vi "PV Write-Read Core.vi"(4 "error in":errorcluster, 5 "Write data in":string, 7 "VISA session":refnum<visa-resource-name>) -> (0 "error out":errorcluster, 1 "response (data) out":string, 3 "dup VISA session":refnum<visa-resource-name>)   [LabVIEW 2015, in "Pfeiffer Vacuum.lvlib"]
uses:
  Pfeiffer Vacuum.lvlib
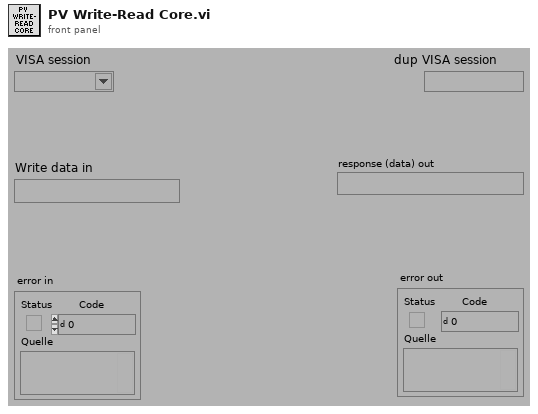
[diagram p1: front panel]
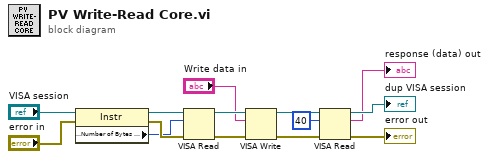
[diagram p0: block diagram]
diagram:
  n1 = property class="Instr"(reference="VISA session", error in="error in") -> (reference out=w11:refnum<visa-resource-name>, error out=w12:errorcluster, "Serial Settings:Number of Bytes at Serial Port"=w10:u32)
  n2 = VISA Read(VISA resource name=w11, byte count=w10, error in (no error)=w12) -> (VISA resource name out=w13:refnum<visa-resource-name>, error out=w5:errorcluster)  [unwired: 2 out]
  n3 = VISA Write(VISA resource name=w13, write buffer="Write data in", error in (no error)=w5) -> (VISA resource name out=w6:refnum<visa-resource-name>, error out=w4:errorcluster)  [unwired: 1 out]
  n4 = VISA Read(VISA resource name=w6, byte count=u32 40 ("Anzahl der Bytes (0)"), error in (no error)=w4) -> (VISA resource name out=→"dup VISA session":refnum<visa-resource-name>, read buffer=→"response (data) out":string, error out=→"error out":errorcluster)  [unwired: 1 out]
